vi "Formula_Node_Ejercicio.vi"() -> ()   [LabVIEW 2020]
panel:
  out "XY Graph":cluster{dbl[], dbl[]}(graph)
  out "Waveform Graph":dbl[](graph)
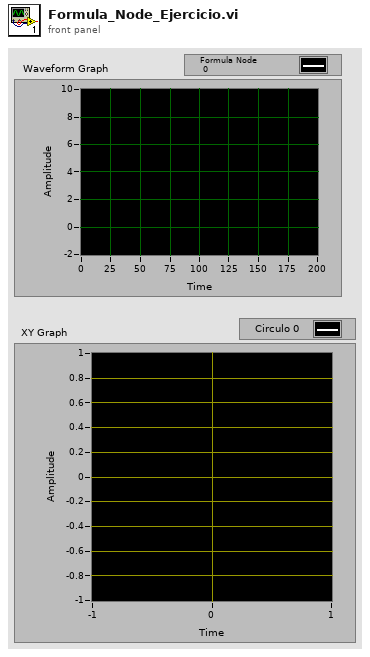
[diagram p1: front panel]
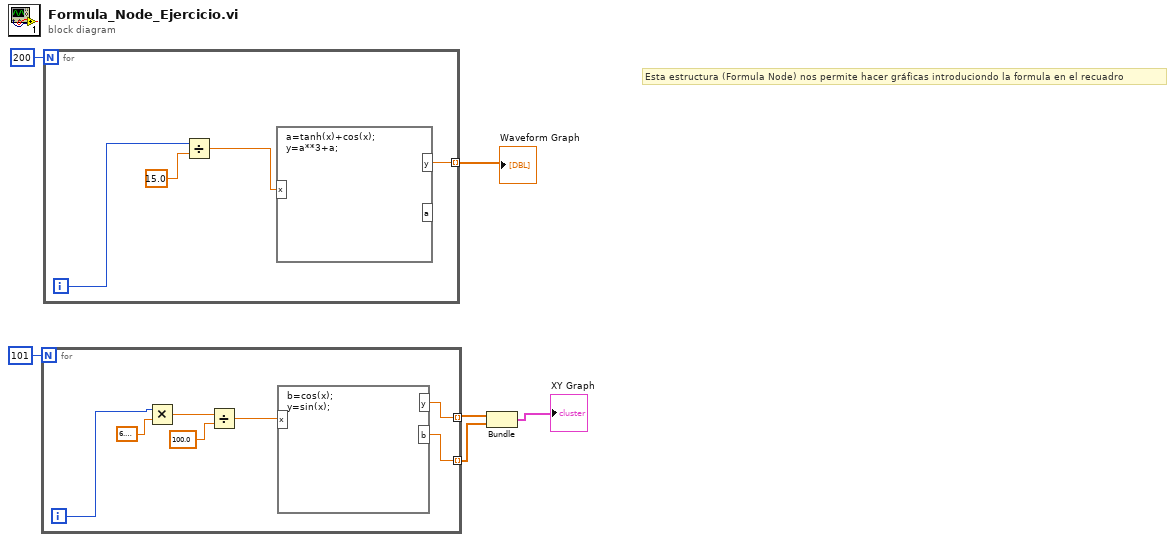
[diagram p0: block diagram]
diagram:
  # "Esta estructura (Formula Node) nos permite hacer gráficas introduciondo la formula en el recuadro"
  n1 = for {
    N: 101 -> [_]
    tunnel: [w8] -> w3 mode=indexing
    tunnel: [w7] -> w2 mode=indexing
    i -> [w12]
    n2 = Multiply(x=w12, y=6.283185307179586) -> (x*y=w11:dbl)
    n3 = Divide(x=w11, y=100.0) -> (x/y=w9:dbl)
    n4 = formula code="b=cos(x);\ny=sin(x);"("x"=w9) -> ("y"=w8:dbl, "b"=w7:dbl)
  }
  n5 = for {
    N: 200 -> [_]
    tunnel: [w14] -> w5 mode=indexing
    i -> [w15]
    n6 = Divide(x=w15, y=15.0) -> (x/y=w17:dbl)
    n7 = formula code="a=tanh(x)+cos(x);\ny=a**3+a;"("x"=w17) -> ("y"=w14:dbl)  [unwired: 1 out]
  }
  "Waveform Graph" <- w5
  n8 = Bundle(w3, w2) -> (→"XY Graph":cluster{dbl[], dbl[]})  [unwired: 1 in]
